vi "StateTransitionEdge_GetObjectStatus.vi"(0 "reference in":refnum<class "StateTransitionEdge.lvclass">, 5 "error in (no error)":errorcluster) -> (10 "# of objects":i32, 11 "Not a refnum?":bool, 12 "All objects names":string[](array[string]), 13 "Class name":string, 14 "reference out":refnum<class "StateTransitionEdge.lvclass">, 15 "Object name":string, 16 "All refs out":refnum<class "StateTransitionEdge.lvclass">[](array[class]), 19 "error out":errorcluster)   [LabVIEW 2016, in "StateTransitionEdge.lvclass"]
doc: "Returns the object status and also information about all the objects in the class."
uses:
  <resource>/Framework/Providers/Open_GDS/UML/StateTransitionEdge_class/StateTransitionEdge.lvclass
  <resource>/Framework/Providers/Open_GDS/UML/StateTransitionEdge_class/protected/ObjectAttributes.ctl
panel:
  in  "DebuggerInput":variant
  out "DebuggerOutput":variant
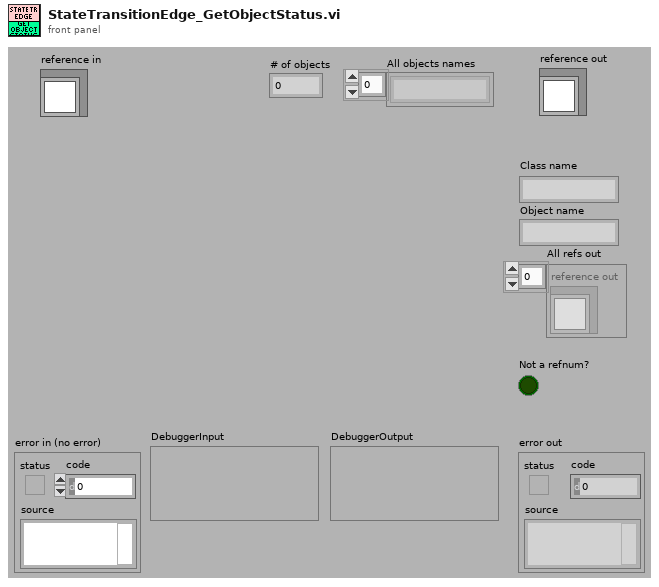
[diagram p1: front panel]
types:
  T1 = typedef "StateTransitionEdge.lvclass/ObjectAttributes.ctl" = cluster{"angle":dbl}
  T2 = cluster{"Mode":enum16{"Get", "Set", "Delete"}, "Ref":variant, "ObjAttribute":string, "ClassAttribute":string}
  T3 = cluster{"Object names":string[], "Refs":variant, "ObjectAttributeLocked":bool, "ClassAttributeLocked":bool, "ObjAttribute":variant, "ClassAttribute":variant}
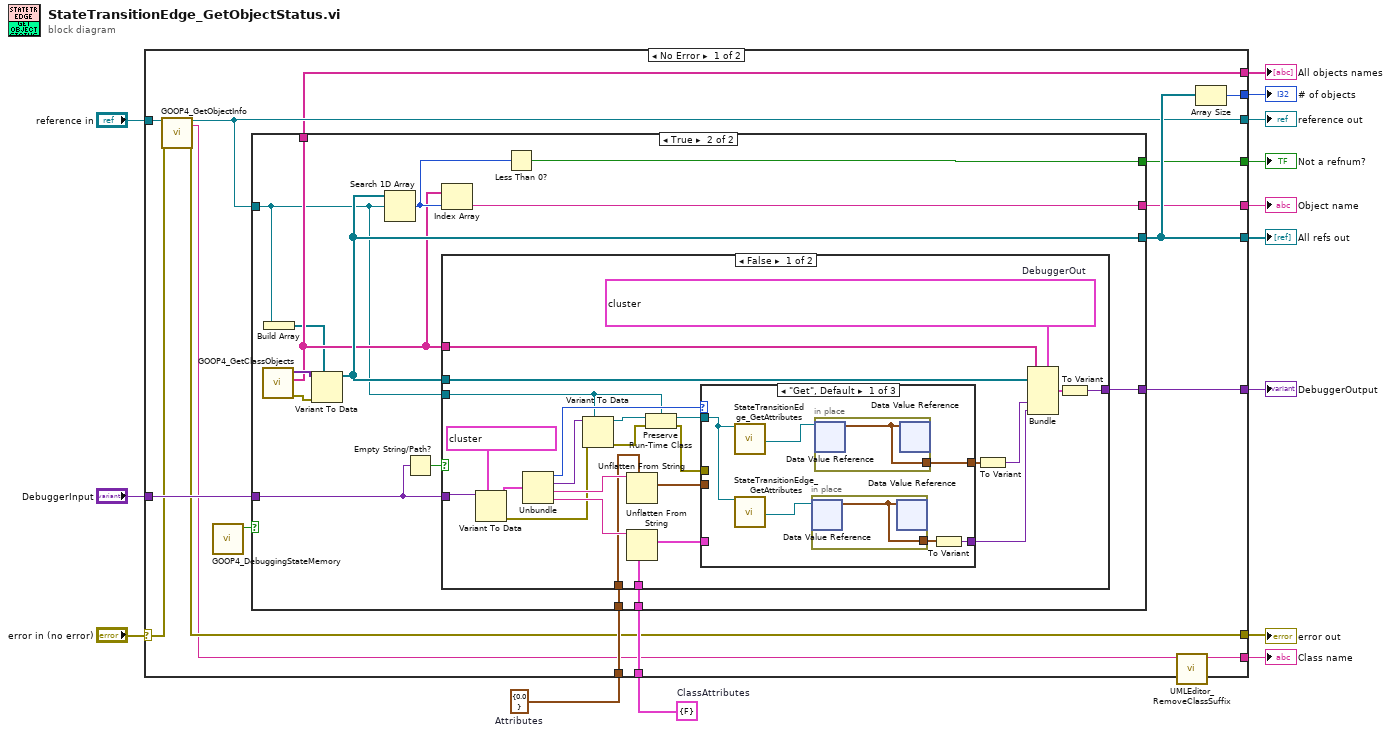
[diagram p0: block diagram]
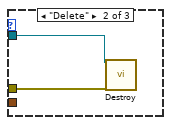
[diagram p3: hidden frame]
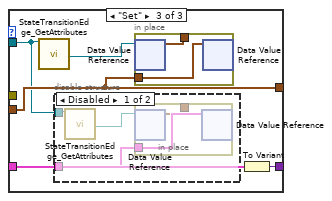
[diagram p4: hidden frame]
diagram:
  w2 = cluster{"classAttribute1":bool} {"classAttribute1"=FALSE}  # ClassAttributes
  w3 = T1 {"angle"=0.0}  # Attributes
  n1 = case shown="No Error" "error in (no error)" {
    selector: "error in (no error)" -> [w26 w92]
    tunnel: "reference in" -> [w28 w96]
    tunnel: [w21 w96] -> w12
    tunnel: [w30 -1 ("# of objects")] -> w1
    tunnel: [w19 TRUE ("Exists?")] -> w11
    tunnel: [w15 w93] -> w10
    tunnel: [w17 string[] [] ("Object names")] -> w9
    tunnel: [w20 w93] -> w8
    tunnel: "DebuggerInput" -> [w27 _]
    tunnel: [w29 _] -> w6
    tunnel: [w23 _] -> w5
    tunnel: w3 -> [w25 _]
    tunnel: w2 -> [w24 _]
    tunnel: [w18 w92] -> w4
    frame No Error {
      n2 = call <vilib>:"GOOP4_GetObjectInfo.vi"("ObjectIn"=w28, "error in (no error)"=w26) -> ("ObjectOut"=w21:refnum<class "StateTransitionEdge.lvclass">, "ObjectRuntimeClassName"=w16:string, "error out"=w18:errorcluster)  [unwired: 12 in, 3 out]
      n3 = call <vilib>:"GOOP4_DebuggingStateMemory.vi"() -> ("CurrentDebuggingState"=w22:bool)  [unwired: 10 in, 1 out]
      n4 = case shown="True" w22 {
        tunnel: w27 -> [_ w43]
        tunnel: [_ w42] -> w29
        tunnel: w25 -> [_ w41]
        tunnel: w24 -> [_ w40]
        tunnel: [_ w35] -> w23
        tunnel: [_ w33] -> w17
        tunnel: w21 -> [_ w32]
        tunnel: [_ w37] -> w20
        tunnel: [_ w36] -> w19
        frame False {
        }
        frame True {
          n5 = call <vilib>:"GOOP4_GetClassObjects.vi"() -> ("error out"=w38:errorcluster, "ObjectNames"=w33:string[], "ObjectsRefs"=w39:variant[])  [unwired: 9 in]
          n6 = Build Array(w32) -> (w31:refnum<class "StateTransitionEdge.lvclass">[])
          n7 = Variant To Data(error in=w38, type=w31, Variant=w39) -> (data=w35:refnum<class "StateTransitionEdge.lvclass">[])  [unwired: 1 out]
          n8 = Search 1D Array(1D array=w35, element=w32) -> (index of element=w34:i32)  [unwired: 1 in]
          n9 = Empty String/Path?(string/path=w43) -> (empty?=w44:bool)
          n10 = Index Array(array=w33, index=w34) -> (element=w37:string)
          n11 = case shown="False" w44 {
            tunnel: [w46 _] -> w42
            tunnel: w41 -> [w66 _]
            tunnel: w40 -> [w65 _]
            tunnel: w43 -> [w58 _]
            tunnel: w35 -> [w54 _]
            tunnel: w33 -> [w60 _]
            tunnel: w32 -> [w53 _]
            frame False {
              w59 = T3 {"Object names"=[], "Refs"=variant, "ObjectAttributeLocked"=FALSE, "ClassAttributeLocked"=FALSE, "ObjAttribute"=variant, "ClassAttribute"=variant}  # DebuggerOut
              n12 = Variant To Data(type=T2 {"Mode"=enum."Delete", "Ref"=variant, "ObjAttribute"="", "ClassAttribute"=""} ("DebuggerIn"), Variant=w58) -> (data=w56:T2, error out=w48:errorcluster)  [unwired: 1 in]
              n13 = Unbundle(w56) -> ("Mode"=w64:enum16{"Get", "Set", "Delete"}, "Ref"=w55:variant, "ObjAttribute"=w68:string, "ClassAttribute"=w69:string)
              n14 = Variant To Data(error in=w48, type=w53, Variant=w55) -> (data=w52:refnum<class "StateTransitionEdge.lvclass">, error out=w50:errorcluster)
              n15 = Unflatten From String(type=w66, binary string=w68) -> (value=w67:T1)  [unwired: 3 in, 2 out]
              n16 = Unflatten From String(type=w65, binary string=w69) -> (value=w63:cluster{"classAttribute1":bool})  [unwired: 3 in, 2 out]
              n17 = Preserve Run-Time Class(object in=w52, error in=w50, 2:w53) -> (object out=w51:refnum<class "StateTransitionEdge.lvclass">, error out=w49:errorcluster)
              n18 = case shown="\"Get\", Default" w64 {
                tunnel: w51 -> [w73 w79 w80]
                tunnel: [w75 _ w83] -> w61
                tunnel: [w70 _ w82] -> w45
                tunnel: w67 -> [_ _ w83]
                tunnel: w63 -> [_ _ w81]
                tunnel: w49 -> [_ w78 _]
                frame "Get", Default {
                  n19 = call <resource>:"StateTransitionEdge_GetAttributes.vi"("reference in"=w73) -> ("DataRef"=w74:refnum<data-value>)  [unwired: 15 in, 3 out]
                  n20 = call <resource>:"StateTransitionEdge_GetAttributes.vi"("reference in"=w73) -> ("DataRef"=w72:refnum<data-value>)  [unwired: 15 in, 3 out]
                  n21 = in-place {
                    in-place-border: [w76] -> w71
                    n22 = in-place-dvr #1(w72) -> (w76:T1)  [unwired: 1 out]
                    n23 = in-place-dvr #1(w76) -> ()  [unwired: 2 out]
                  }
                  n24 = in-place {
                    in-place-border: [w77] -> w75
                    n25 = in-place-dvr #2(w74) -> (w77:T1)  [unwired: 1 out]
                    n26 = in-place-dvr #2(w77) -> ()  [unwired: 2 out]
                  }
                  n27 = To Variant(anything=w71) -> (Variant=w70:variant)
                }
                frame "Delete" {
                  n28 = call-dynamic "Destroy.vi"("reference"=w79, "error in (no error)"=w78) -> ()  [unwired: 17 in, 1 out]
                }
                frame "Set" {
                  n29 = call <resource>:"StateTransitionEdge_GetAttributes.vi"("reference in"=w80) -> ("DataRef"=w84:refnum<data-value>)  [unwired: 15 in, 3 out]
                  n30 = disable-structure shown="Disabled" {
                    disable-tunnel: w81 -> [w86 _]
                    disable-tunnel: w80 -> [w85 _]
                    frame Disabled {
                      n31 = call <resource>:"StateTransitionEdge_GetAttributes.vi"("reference in"=w85) -> ("DataRef"=w87:refnum<data-value>)  [unwired: 15 in, 3 out]
                      n32 = in-place {
                        in-place-border: w86 -> [w89]
                        in-place-border: [w88] -> _
                        n33 = in-place-dvr #3(w87) -> (w88:T1)  [unwired: 1 out]
                        n34 = in-place-dvr #3(w89) -> ()  [unwired: 2 out]
                      }
                    }
                    frame Enabled {
                    }
                  }
                  n35 = in-place {
                    in-place-border: w83 -> [w91]
                    in-place-border: [w90] -> _
                    n36 = in-place-dvr #4(w84) -> (w90:T1)  [unwired: 1 out]
                    n37 = in-place-dvr #4(w91) -> ()  [unwired: 2 out]
                  }
                  n38 = To Variant(anything=w81) -> (Variant=w82:variant)
                }
              }
              n39 = To Variant(anything=w61) -> (Variant=w62:variant)
              n40 = Bundle(cluster=w59, "Object names"=w60, "Refs"=w54, "ObjAttribute"=w62, "ClassAttribute"=w45) -> (w47:T3)  [unwired: 2 in]
              n41 = To Variant(anything=w47) -> (Variant=w46:variant)
            }
            frame True {
            }
          }
          n42 = Less Than 0?(x=w34) -> (x < 0?=w36:bool)
        }
      }
      n43 = call <resource>:"UMLEditor_RemoveClassSuffix.vi"("ObjectRuntimeClassName in"=w16) -> ("ObjectRuntimeClassName out"=w15:string)  [unwired: 10 in]
      n44 = Array Size(array=w23) -> (size(s)=w30:i32)
    }
    frame Error {
      w93 = "" ("Class name")
      (unwired) FALSE
    }
  }
  "error out" <- w4
  "reference out" <- w12
  "# of objects" <- w1
  "Not a refnum?" <- w11
  "All refs out" <- w5
  "Class name" <- w10
  "All objects names" <- w9
  "Object name" <- w8
  "DebuggerOutput" <- w6
